vi "starast.vi"() -> ()   [LabVIEW 2010]
panel:
  in  "CRPIX2":dbl
  in  "CRPIX1":dbl
  in  "CRVAL2":dbl
  in  "CRVAL1":dbl
  in  "secperpulse":dbl
  out "CD":dbl[][](array[numeric])
  in  "Y":dbl[](array[numeric])
  in  "X":dbl[](array[numeric])
  in  "DEC":dbl[](array[numeric])
  in  "RA":dbl[](array[numeric])
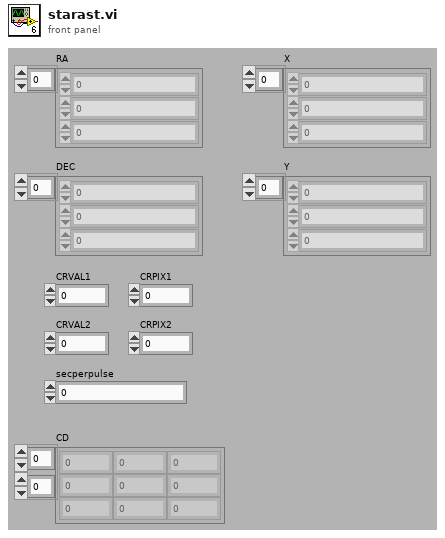
[diagram p1: front panel]
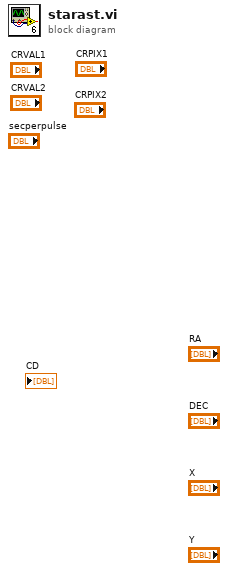
[diagram p0: block diagram]
diagram:
